vi "exercise7_readAI_samplesloop.vi"() -> ()   [LabVIEW 2018]
uses:
  <vilib>/DAQmx/read.llb/DAQmx Read (Analog 1D Wfm NChan NSamp).vi
  <vilib>/DAQmx/create/channels.llb/DAQmx Create Channel (AI-Voltage-Basic).vi
  <vilib>/DAQmx/configure/timing.llb/DAQmx Timing (Sample Clock).vi
  <vilib>/DAQmx/miscellaneous.llb/DAQmx Fill In Error Info.vi
  <vilib>/express/express analysis/Spectral/Block/exnSpectralBlock spectral measurements RMS poly.vi
  <vilib>/express/express analysis/Spectral/Block/exnSpectralBlock spectral measurements RMS array WFM.vi
  <vilib>/express/express analysis/Spectral/XNode/ExpressSpectralMeasurementsBlockNode.xnode
panel:
  in  "NI_channels 2":tag="Dev1/ai0"
  out "SINAD (dB) - ai1":dbl(knob) scale=0.0..100.0
  out "SINAD (dB) - ai0":dbl(knob) scale=0.0..100.0
  out "Waveform Chart (Pa)":waveform(dbl)[](graph)
  out "FFT":cluster{"f0":dbl, "df":dbl, "magnitude":dbl[]}[](graph)
  in  "?":bool
  in  "maximum value":dbl=5.0
  in  "minimum value":dbl=-5.0
  in  "sample mode":i32(ring)=10123 items=["Finite Samples"=10178, "Continuous Samples"=10123, "Hardware Timed Single Point"=12522]
  in  "samples per channel":i32=40
  in  "rate":dbl=20.0
  out "error out":errorcluster
  out "Waveform Graph":waveform(dbl)[](graph)
  out "Waveform Chart":waveform(dbl)[](graph)
  in  "NI_channels":tag="Dev1/ai0"
  # "CANAL 0"
  # "CANAL 0"
  # "ACQUIRE SIGNAL (CONTINUOUS)"
  # "CHANNEL CONFIG"
  # "SAMPLING CONFIG"
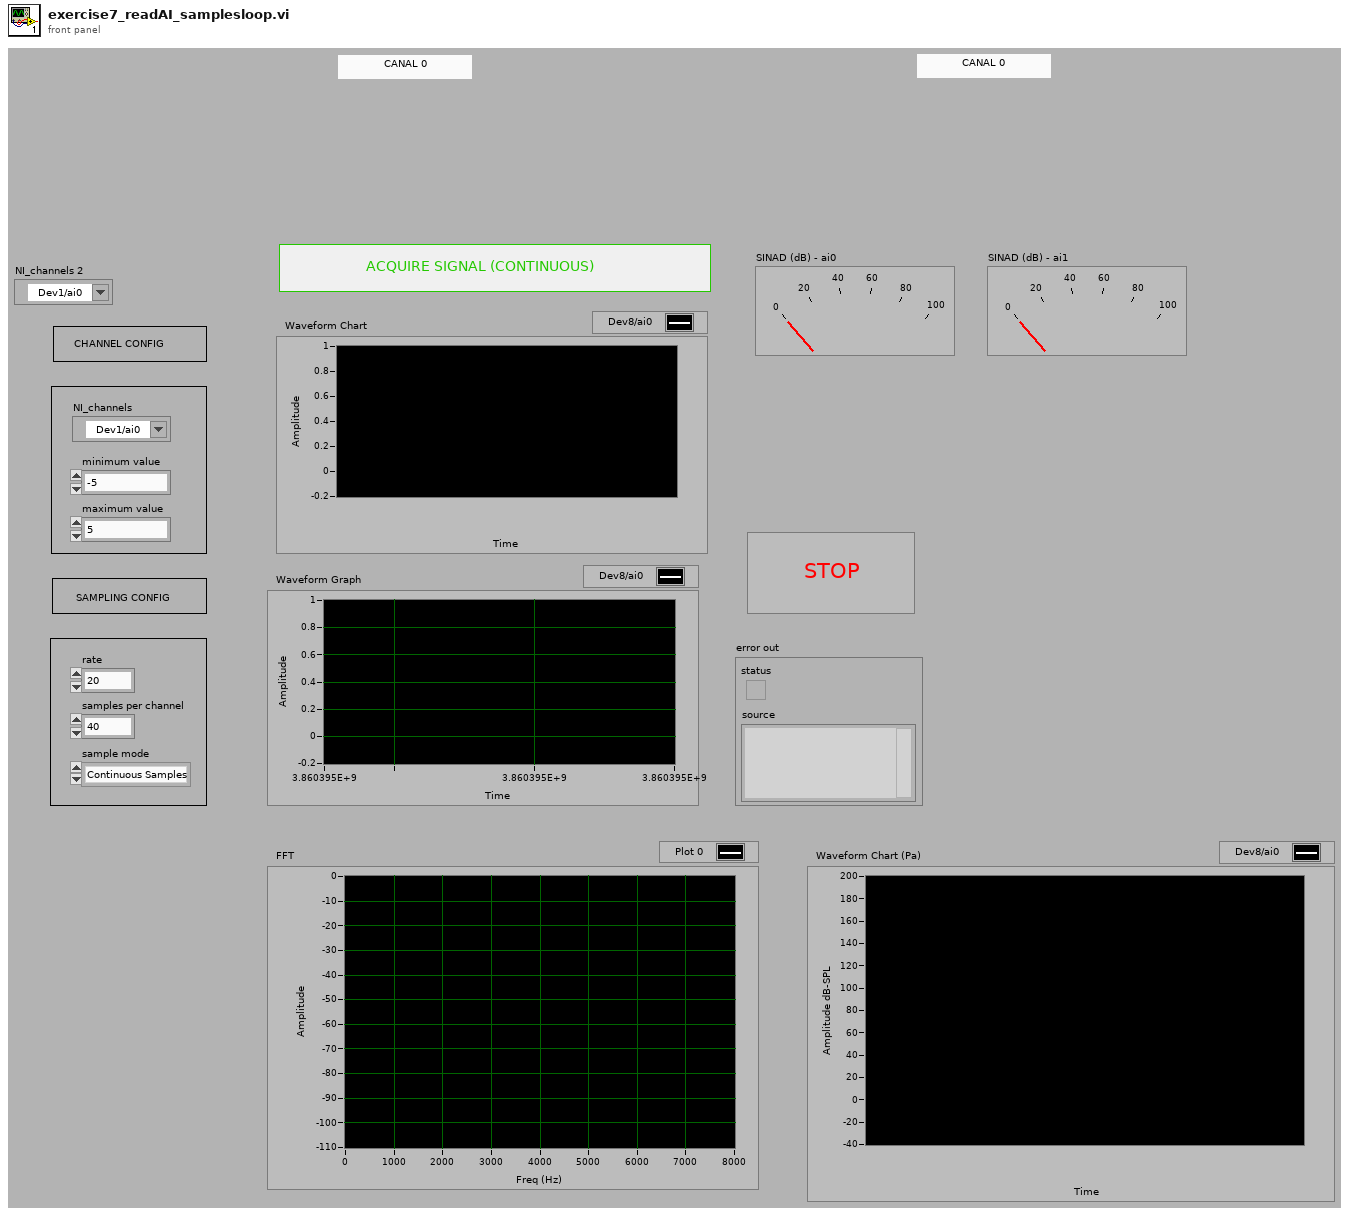
[diagram p1: front panel]
types:
  T1 = cluster{"averaging mode":u16, "weighting mode":u16, "number of averages":u32}
  T2 = cluster{"dB On (F)":bool, "unwrap phase (F)":bool, "convert to degree (F)":bool}
  T3 = cluster{"data[0]":waveform(dbl), "data[1]":waveform(dbl), "data[2]":waveform(dbl), "data[3]":waveform(dbl), "data[4]":waveform(dbl), "data[5]":waveform(dbl), "data[6]":waveform(dbl), "data[7]":waveform(dbl), "data[8]":waveform(dbl)}
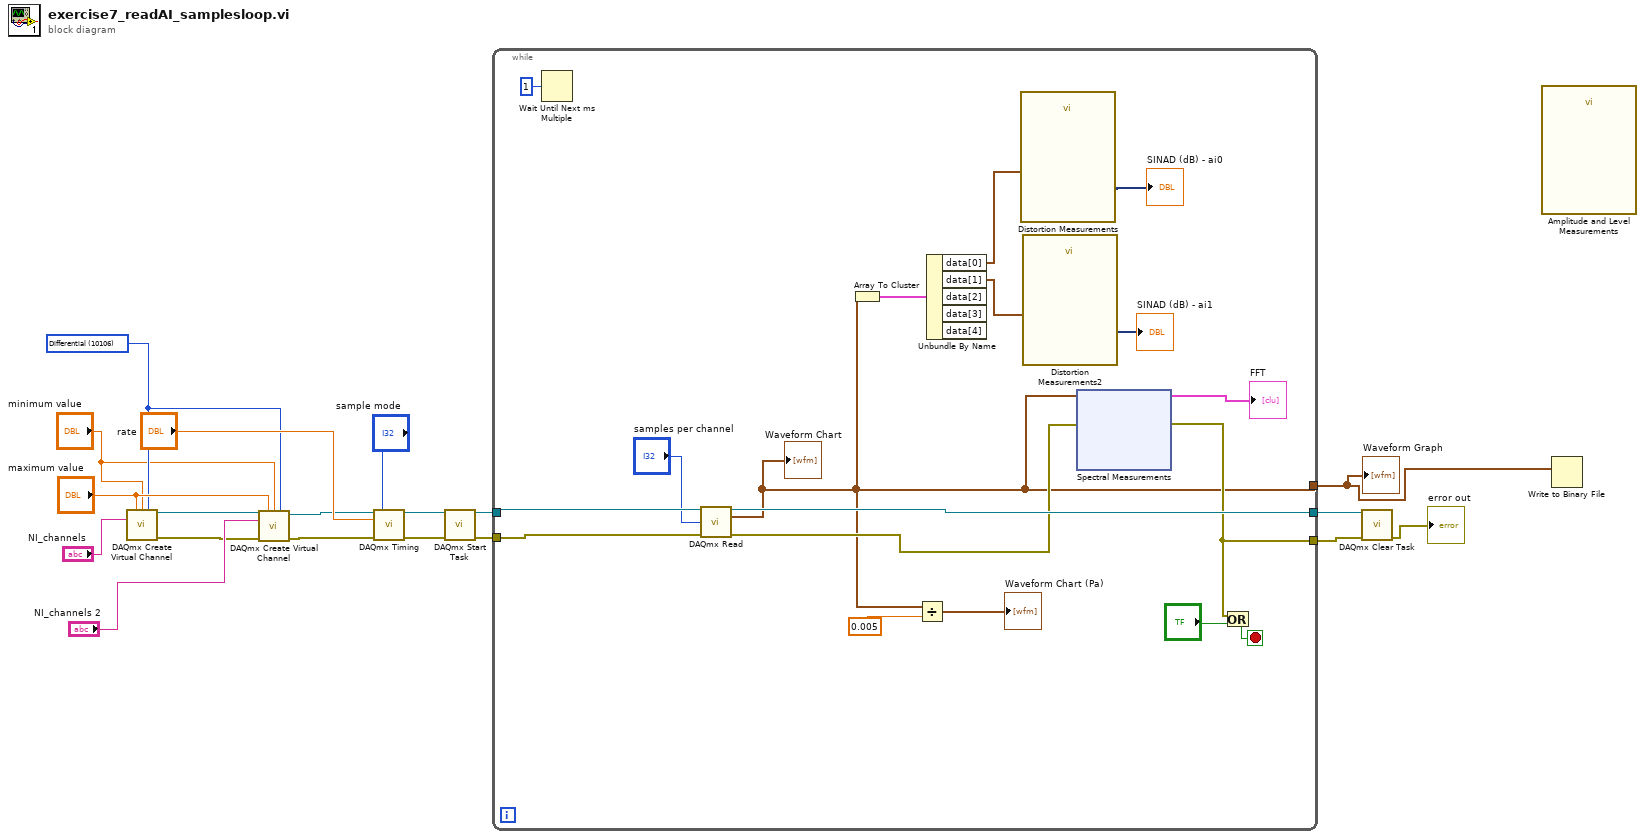
[diagram p0: block diagram]
diagram:
  w5 = 10106 items=["default"=-1, "RSE"=10083, "NRSE"=10078, "Differential"=10106, "Pseudodifferential"=12529] ("input terminal configuration")
  n1 = call-poly <vilib>:"DAQmx Create Virtual Channel.vi"("maximum value"="maximum value", "minimum value"="minimum value", "input terminal configuration"=w5, "physical channels"="NI_channels") -> ("task out"=w8:refnum<k21>, "error out"=w2:errorcluster)  [unwired: 10 in]
  n2 = call-poly <vilib>:"DAQmx Create Virtual Channel.vi"("task in"=w8, "maximum value"="maximum value", "minimum value"="minimum value", "input terminal configuration"=w5, "physical channels"="NI_channels 2", "error in"=w2) -> ("task out"=w7:refnum<k21>, "error out"=w1:errorcluster)  [unwired: 8 in]
  n3 = call-poly <vilib>:"DAQmx Timing.vi"("task/channels in"=w7, "sample mode"="sample mode", "rate"="rate", "error in"=w1) -> ("task out"=w16:refnum<k21>, "error out"=w15:errorcluster)  [unwired: 10 in]
  n4 = call <vilib>:"DAQmx Start Task.vi"("task/channels in"=w16, "error in"=w15) -> ("task out"=w13:refnum<k21>, "error out"=w14:errorcluster)  [unwired: 12 in]
  n5 = while {
    tunnel: w14 -> [w37]
    tunnel: w13 -> [w36]
    tunnel: [w25] -> w9
    tunnel: [w35] -> w12
    tunnel: [w28] -> w11
    stop <- w32 stop-if-true
    n6 = Wait Until Next ms Multiple(millisecond multiple=u32 1) -> ()  [unwired: 1 out]
    n7 = call-poly <vilib>:"DAQmx Read.vi"("task/channels in"=w36, "number of samples per channel"="samples per channel", "error in"=w37) -> ("task out"=w35:refnum<k21>, "data"=w25:waveform(dbl)[], "error out"=w29:errorcluster)  [unwired: 10 in]
    "Waveform Chart" <- w25
    n8 = Array To Cluster(array=w25) -> (cluster=w24:T3)
    n9 = Divide(x=w25, y=0.005) -> (x/y=→"Waveform Chart (Pa)":waveform(dbl)[])
    n10 = Unbundle By Name "Unbundle By Name"(w24) -> ("data[0]"=w22:waveform(dbl), "data[1]"=w20:waveform(dbl))  [unwired: 3 out]
    n11 = call "Distortion Measurements"("Signals"=w22) -> ("SINAD (dB)"=→"SINAD (dB) - ai0":dynamicdata)  [unwired: 8 in, 2 out]
    n12 = call "Distortion Measurements2"("Signals"=w20) -> ("SINAD (dB)"=→"SINAD (dB) - ai1":dynamicdata)  [unwired: 8 in, 2 out]
    n13 = xnode "Spectral Measurements"("Signals"=w25, "error in (no error)"=w29) -> ("FFT - (RMS)"=→"FFT":cluster{"f0":dbl, "df":dbl, "magnitude":dbl[]}[], "error out"=w28:errorcluster)  [unwired: 1 out]
    n14 = Or(x=w28, y="?") -> (x .or. y?=w32:bool)
  }
  "Waveform Graph" <- w9
  n15 = call <vilib>:"DAQmx Clear Task.vi"("task in"=w12, "error in"=w11) -> ("error out"=→"error out":errorcluster)  [unwired: 13 in]
  n16 = call "Amplitude and Level Measurements"() -> ()  [unwired: 14 in, 2 out]
  n17 = Write to Binary File(data=w9) -> ()  [unwired: 5 in, 3 out]
